vi "Set Remote Terminal Endpoint.vi"(8 "error in":errorcluster, 9 "direction":T1, 10 "remote terminal":T2, 11 "message in":T4 format="%.0x") -> (0 "error out":errorcluster, 3 "message out":T4 format="%.0x")   [LabVIEW 2020, in "AIM MIL-STD-1553 Scripting.lvlib"]
doc: "Sets remote terminal address and subaddress properties on the message. The properties are namespaced by input direction."
uses:
  AIM MIL-STD-1553 Scripting.lvlib
  Constants.vi
  <vilib>/NI VeriStand/Custom Device API/Custom Device API.lvlib
  <vilib>/NI VeriStand/Custom Device API/Set Item Property (U16).vi
  <vilib>/NI VeriStand/Custom Device API/Custom Device Item Ref.ctl
  Shared/Address.ctl
  Shared/Terminal Endpoint.ctl
  Shared/Direction.ctl
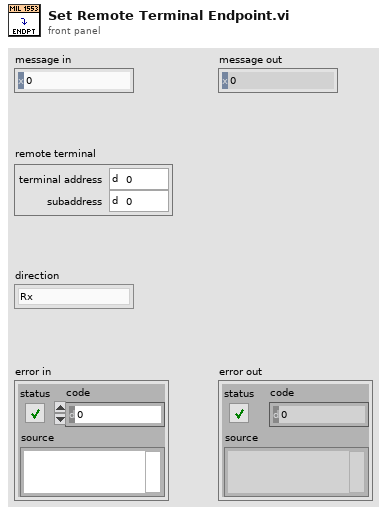
[diagram p1: front panel]
types:
  T1 = typedef "Direction.ctl" = enum16{"Rx", "Tx"}
  T2 = typedef "Terminal Endpoint.ctl" = cluster{"terminal address":T3, "subaddress":T3}
  T3 = typedef "Address.ctl" = u16
  T4 = typedef "Custom Device API.lvlib/Custom Device Item Ref.ctl" = u64
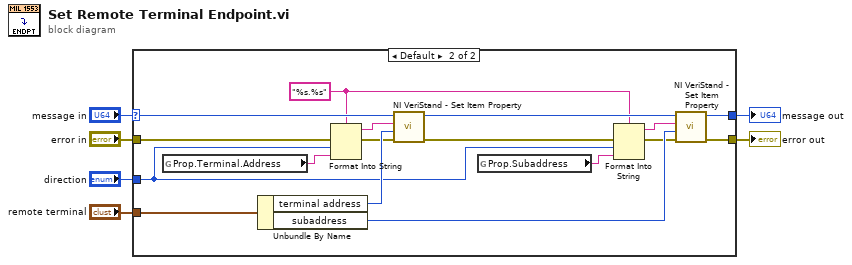
[diagram p0: block diagram]
diagram:
  n1 = case shown="Default" "message in" {
    selector: "message in" -> [w8 w24]
    tunnel: "remote terminal" -> [_ w25]
    tunnel: [w8 w22] -> w4
    tunnel: "direction" -> [_ w14]
    tunnel: "error in" -> [w7 w17]
    tunnel: [w7 w21] -> w1
    frame 0, -1 {
    }
    frame Default {
      w9 = "%s.%s" ("format string")
      n2 = global read "Constants.vi" "Prop.Terminal.Address"() -> (w16:string)
      n3 = Unbundle By Name(w25) -> ("terminal address"=w20:T3, "subaddress"=w19:T3)
      n4 = Format Into String(format string=w9, error in=w17, w14, w16) -> (resulting string=w15:string, error out=w18:errorcluster)  [unwired: 1 in]
      n5 = call-poly <vilib>:"NI VeriStand - Set Item Property.vi"("error in (no error)"=w18, "Value"=w20, "Property Name"=w15, "Item Ref in"=w24) -> ("error out"=w11:errorcluster, "Item Ref out"=w23:T4)  [unwired: 5 in, 1 out]
      n6 = global read "Constants.vi" "Prop.Subaddress"() -> (w13:string)
      n7 = Format Into String(format string=w9, error in=w11, w14, w13) -> (resulting string=w12:string, error out=w10:errorcluster)  [unwired: 1 in]
      n8 = call-poly <vilib>:"NI VeriStand - Set Item Property.vi"("error in (no error)"=w10, "Value"=w19, "Property Name"=w12, "Item Ref in"=w23) -> ("error out"=w21:errorcluster, "Item Ref out"=w22:T4)  [unwired: 5 in, 1 out]
    }
  }
  "message out" <- w4
  "error out" <- w1
